vi "Array Bools to Mapping.vi"(10 "Related is Array":bool, 11 "This is Array":bool) -> (3 "Relation Mapping":T1)   [LabVIEW 2020, in "Conditum-Tools.lvlib" / "RelationPanel.lvclass"]
uses:
  RelationPanel.lvclass
  Conditum-Clone/Relation Mapping.ctl
  Conditum-Clone/Conditu2.lvlib
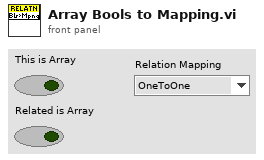
[diagram p1: front panel]
types:
  T1 = typedef "Conditu2.lvlib/Relation Mapping.ctl" = enum16{"OneToOne", "OneToMany", "ManyToOne", "ManyToMany"}
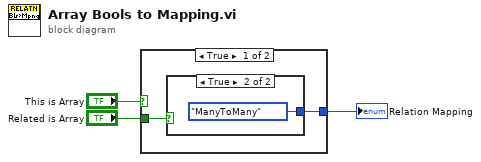
[diagram p0: block diagram]
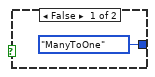
[diagram p2: hidden frame]
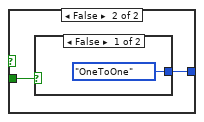
[diagram p3: hidden frame]
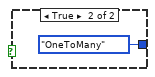
[diagram p4: hidden frame]
diagram:
  n1 = case shown="True" "This is Array" {
    tunnel: "Related is Array" -> [w5 w9]
    tunnel: [w4 w8] -> w1
    frame True {
      n2 = case shown="True" w5 {
        tunnel: [Relation_Mapping."ManyToOne" ("Relation Mapping") Relation_Mapping."ManyToMany" ("Relation Mapping")] -> w4
        frame False {
        }
        frame True {
        }
      }
    }
    frame False {
      n3 = case shown="False" w9 {
        tunnel: [Relation_Mapping."OneToOne" ("Relation Mapping") Relation_Mapping."OneToMany" ("Relation Mapping")] -> w8
        frame False {
        }
        frame True {
        }
      }
    }
  }
  "Relation Mapping" <- w1
